vi "NI VeriStand - Wait For Macro Player Completion.vi"(8 "error in (no error)":errorcluster, 11 "MacroPlayer in":T1) -> (0 "error out":errorcluster, 3 "MacroPlayer out":T1)   [LabVIEW 2020, in "NI_VS MacroPlayerAPI.lvlib"]
doc: "Waits for the Macro Player tool to finish playing back the current macro file before continuing execution and returning a reference to the Macro Player."
uses:
  <vilib>/NI VeriStand/Execution/MacroPlayer/NI_VS MacroPlayerAPI.lvlib
  <vilib>/NI VeriStand/Execution/MacroPlayer/MacroPlayerAPI.ctl
  NationalInstruments.VeriStand.ClientAPI
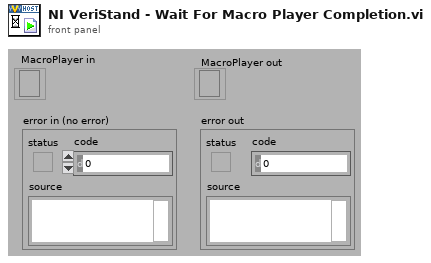
[diagram p1: front panel]
types:
  T1 = typedef "NI_VS MacroPlayerAPI.lvlib/MacroPlayerAPI.ctl" = refnum<k24>
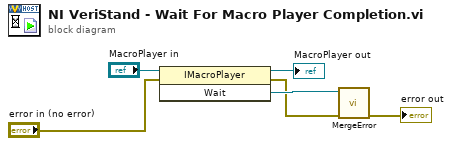
[diagram p0: block diagram]
diagram:
  n1 = invoke class="IMacroPlayer" method="Wait"(reference="MacroPlayer in", error in="error in (no error)") -> (reference out=→"MacroPlayer out":T1, error out=w2:errorcluster, "Wait"=w3:refnum<k24>)  [unwired: 1 in]
  n2 = call <vilib>:"MergeError.vi"("error in (no error)"=w2, "Error"=w3) -> ("error out"=→"error out":errorcluster)  [unwired: 9 out]
